vi "ConfigureSampleClock.vi"(7 "enable External Clock":bool, 9 "external Clock Rate (Hz)":dbl=80000000.0 format="%.2p") -> (19 "Error Out":errorcluster)   [LabVIEW 2015]
doc: "Configures device parameters for an NI 5170/5171"
uses:
  <instrlib>/HSAI-RIO/Types/v1/Host/Typedefs/Reference Clock Source.ctl
  <instrlib>/HSAI-RIO/Types/v1/Host/Typedefs/External Clock Source.ctl
  OscopeAPI/Device Session.lvclass
  <instrlib>/HSAI-RIO/Types/v1/Host/niHSAI Types v1 Host.lvlib
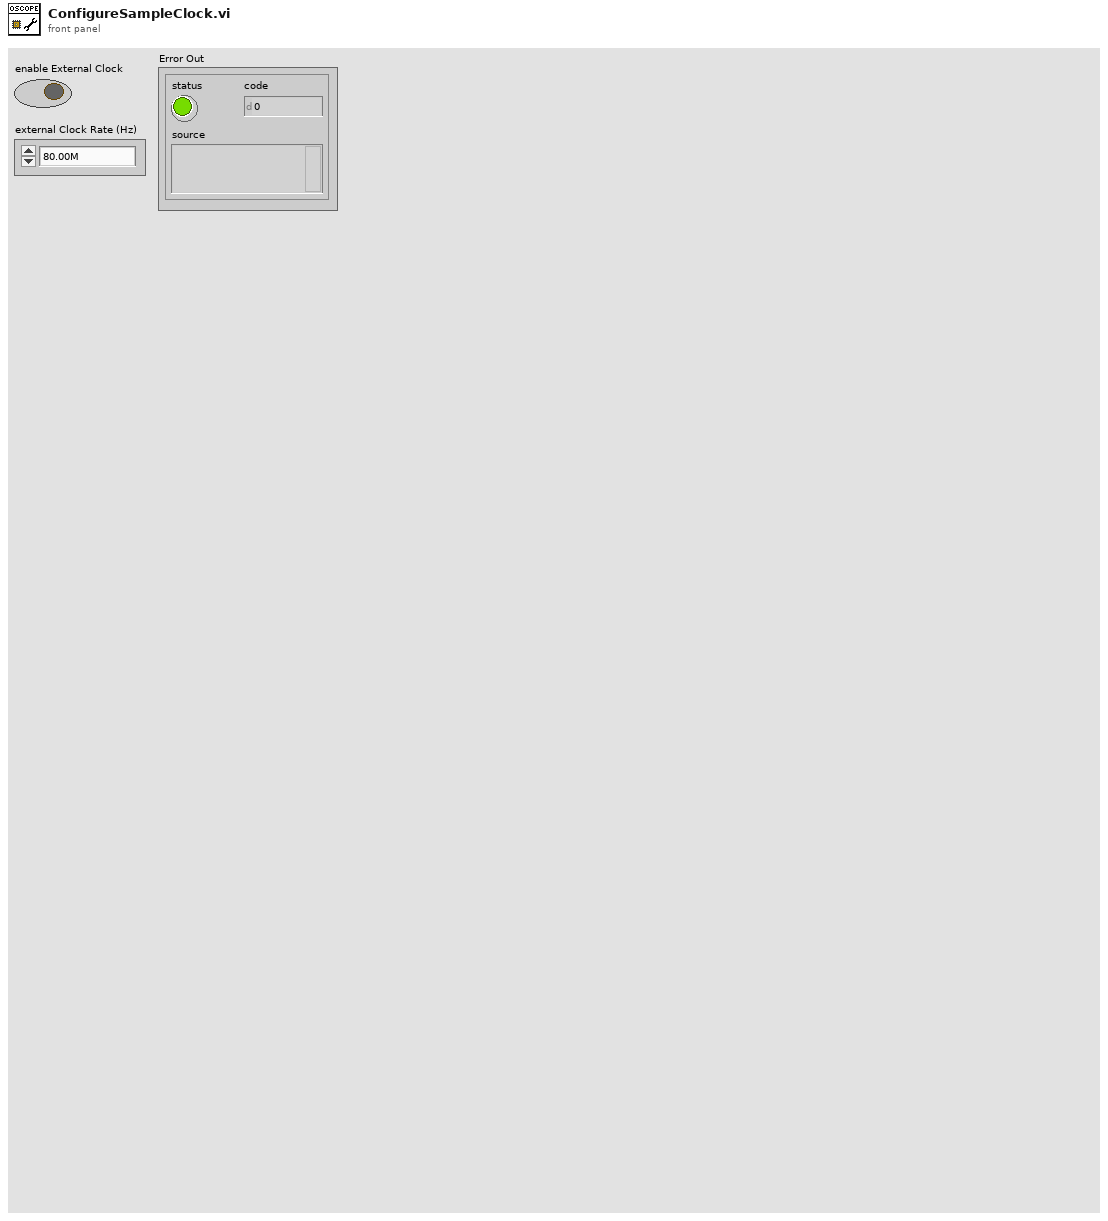
[diagram p1: front panel]
types:
  T1 = typedef "niHSAI Types v1 Host.lvlib/Reference Clock Source.ctl" = enum8{"None", "Clock In", "PXI Clock"}
  T2 = typedef "niHSAI Types v1 Host.lvlib/External Clock Source.ctl" = enum8{"Clock In", "PXIe DStar A"}
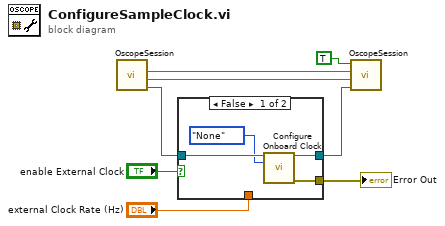
[diagram p0: block diagram]
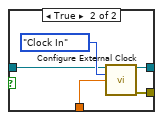
[diagram p2: hidden frame]
diagram:
  n1 = call "OscopeSession.vi"() -> ("Session Out"=w5:refnum<class "Device Session.lvclass">, "Bitfile Path Out"=w2:string, "Device Address Out"=w3:string)  [unwired: 9 in]
  n2 = case shown="False" "enable External Clock" {
    tunnel: w5 -> [w12 w16]
    tunnel: "external Clock Rate (Hz)" -> [_ w15]
    tunnel: [w11 w14] -> w1
    tunnel: [w10 w13] -> w4
    frame False {
      n3 = call "Configure Onboard Clock.vi"("device session in"=w12, "reference clock source"=Reference_Clock_Source."None") -> ("device session out"=w11:refnum<class "Device Session.lvclass">, "error out"=w10:errorcluster)  [unwired: 10 in, 2 out]
    }
    frame True {
      n4 = call "Configure External Clock.vi"("device session in"=w16, "external clock source"=External_Clock_Source."Clock In", "external clock rate (Hz)"=w15) -> ("device session out"=w14:refnum<class "Device Session.lvclass">, "error out"=w13:errorcluster)  [unwired: 10 in, 1 out]
    }
  }
  "Error Out" <- w4
  n5 = call "OscopeSession.vi"("Session In"=w1, "Bitfile Path In"=w2, "Device Address In"=w3, "Write"=TRUE) -> ()  [unwired: 5 in, 3 out]
